vi "Stand Alone UI Initialize.vi"(8 "error in (no error)":errorcluster, 11 "Stand Alone Display Actor in":refnum<class "Stand Alone Display Actor.lvclass">) -> (0 "error out":errorcluster, 3 "Stand Alone Display Actor out":refnum<class "Stand Alone Display Actor.lvclass">)   [LabVIEW 2024, in "Stand Alone Display Actor.lvclass"]
uses:
  Stand Alone Display Actor.lvclass
  Stand Alone Display Actor.lvclass/Stand Alone Display Actor.ctl
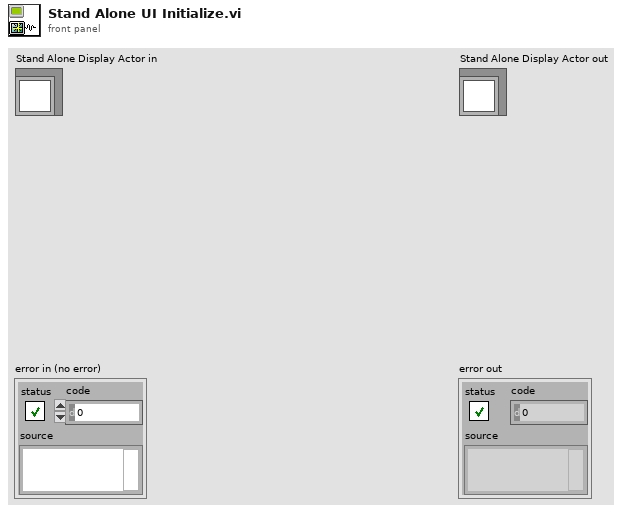
[diagram p1: front panel]
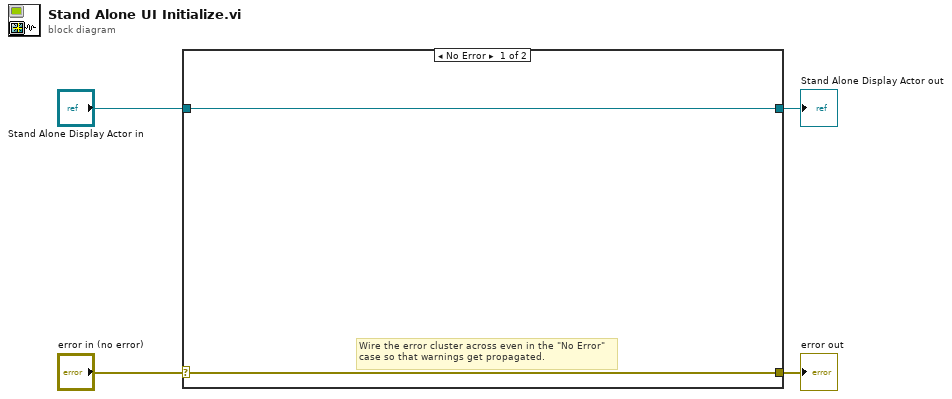
[diagram p0: block diagram]
diagram:
  n1 = case shown="No Error" "error in (no error)" {
    selector: "error in (no error)" -> [w5 w8]
    tunnel: [w5 w8] -> w3
    tunnel: [w6 w7] -> w1
    tunnel: "Stand Alone Display Actor in" -> [w6 w7]
    frame No Error {
      # "Wire the error cluster across even in the \"No Error\"\ncase so that warnings get propagated."
    }
    frame Error {
    }
  }
  "error out" <- w3
  "Stand Alone Display Actor out" <- w1
